vi "ReadState.vi"(8 "Error In":errorcluster, 11 "object in":refnum<class "Flipflop.lvclass">) -> (0 "Error Out":errorcluster, 2 "State":bool, 3 "object out":refnum<class "Flipflop.lvclass">)   [LabVIEW 2021, in "Flipflop.lvclass"]
uses:
  Flipflop.lvclass
  Flipflop.lvclass/Flipflop.ctl
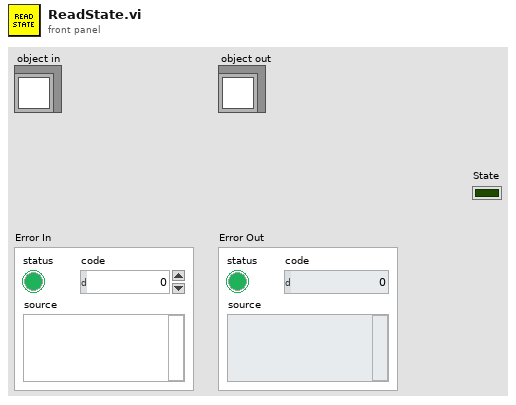
[diagram p1: front panel]
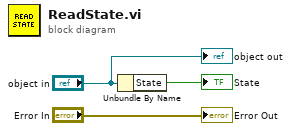
[diagram p0: block diagram]
diagram:
  n1 = Unbundle By Name("object in") -> ("State"=→"State":bool)
  "Error Out" <- "Error In"
  "object out" <- "object in"
